vi "GetMPOR.vi"(10 "全部信号数组":string[][](array[string]), 11 "当前信号":string[](array[string])) -> (3 "MPOR":string[](array[string]))   [LabVIEW 2015]
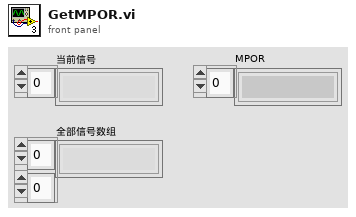
[diagram p1: front panel]
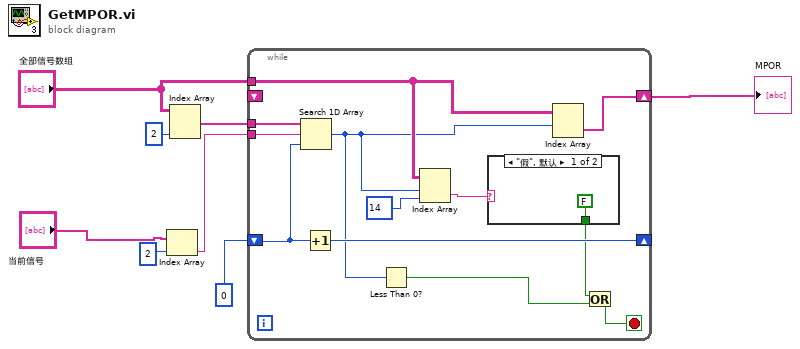
[diagram p0: block diagram]
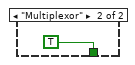
[diagram p2: hidden frame]
diagram:
  n1 = Index Array(array="当前信号", index=2 ("禁用的索引 (列)")) -> (element=w8:string)
  n2 = Index Array(array="全部信号数组", index (col)=2 ("禁用的索引 (列)")) -> (element=w5:string[])  [unwired: 1 in]
  n3 = while {
    tunnel: w8 -> [w20]
    tunnel: w5 -> [w19]
    tunnel: "全部信号数组" -> [w15]
    shift-right: [w16] -> _
    shift-left: 0 -> [w17]
    shift-right: [w18] -> w4
    shift-left: _ -> [_]
    stop <- w9 stop-if-true
    n4 = Search 1D Array(1D array=w19, element=w20, start index (0)=w17) -> (index of element=w12:i32)
    n5 = Increment(x=w17) -> (x+1=w16:i32)
    n6 = Less Than 0?(x=w12) -> (x < 0?=w10:bool)
    n7 = Index Array(array=w15, index (row)=w12, index (col)=14 ("禁用的索引 (列)")) -> (element=w13:string)
    n8 = case shown="\"假\", 默认" w13 {
      tunnel: [FALSE TRUE] -> w11
      frame "假", Default {
      }
      frame "Multiplexor" {
      }
    }
    n9 = Index Array(array=w15, index (row)=w12) -> (element=w18:string[])  [unwired: 1 in]
    n10 = Or(x=w11, y=w10) -> (x .or. y?=w9:bool)
  }
  "MPOR" <- w4
